vi "Configure Linear Math Calculation.vi"(7 "Units (MX)":string="MX", 8 "error in (no error)":errorcluster, 9 "Offset Value (0)":dbl, 10 "Scale Factor (1)":dbl=1.0, 11 "VISA resource name":refnum<visa-resource-name>) -> (0 "error out":errorcluster, 3 "VISA resource name out":refnum<visa-resource-name>)   [LabVIEW 2020, in "Keithley 2182.lvlib"]
doc: "Configures the mX+b math calculation.\n\nThis math operation manipulates normal display readings (X) mathematically according to the following calculation: <B>Y = mX+b</B>\n where:\n <B>X</B> is the normal display reading\n <B>m</B> and <B>b</B> are user-entered constants for scale factor and offset.\n <B>Y</B> is the displayed result"
uses:
  Keithley 2182.lvlib
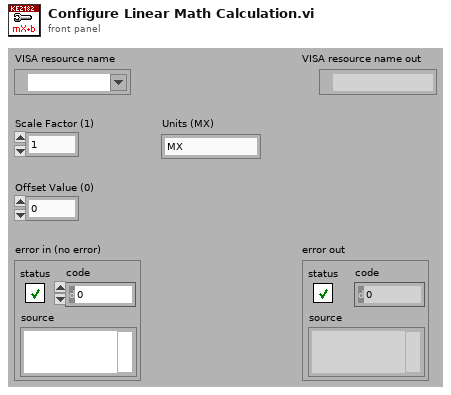
[diagram p1: front panel]
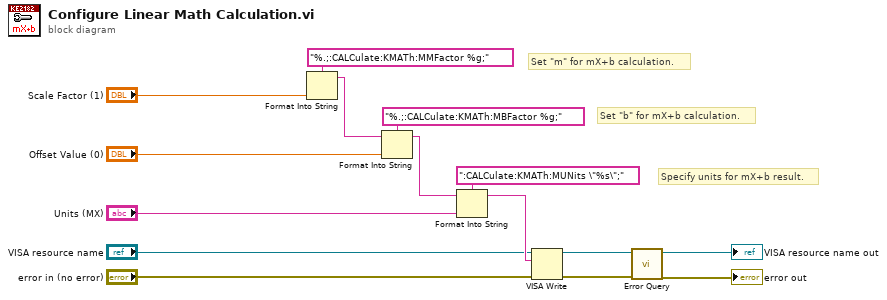
[diagram p0: block diagram]
diagram:
  # "Specify units for mX+b result."
  # "Set \"b\" for mX+b calculation."
  # "Set \"m\" for mX+b calculation."
  n1 = Format Into String(format string="%.;:CALCulate:KMATh:MMFactor %g;", "Scale Factor (1)") -> (resulting string=w13:string)  [unwired: 2 in, 1 out]
  n2 = Format Into String(format string="%.;:CALCulate:KMATh:MBFactor %g;", initial string=w13, "Offset Value (0)") -> (resulting string=w10:string)  [unwired: 1 in, 1 out]
  n3 = Format Into String(format string=":CALCulate:KMATh:MUNits \"%s\";", initial string=w10, "Units (MX)") -> (resulting string=w7:string)  [unwired: 1 in, 1 out]
  n4 = VISA Write(VISA resource name="VISA resource name", write buffer=w7, error in (no error)="error in (no error)") -> (VISA resource name out=w4:refnum<visa-resource-name>, error out=w3:errorcluster)  [unwired: 1 out]
  n5 = call "Error Query.vi"("error in (no error)"=w3, "VISA resource name"=w4) -> ("error out"=→"error out":errorcluster, "VISA resource name out"=→"VISA resource name out":refnum<visa-resource-name>)  [unwired: 6 in, 2 out]
